vi "populateArrays_sub.vi"(11 "Instance":i32) -> (0 "ENC_VEL_Array":u16[](array[numeric]), 1 "ENC_POS_Array":i32[](array[numeric]), 2 "ADC_Array":dbl[](array[numeric]), 3 "Instance out":i32, 4 "DIN":u16, 6 "Message Count":u32)   [LabVIEW 2022 SP3]
uses:
  LVLib/SADI_FW3.lvlib
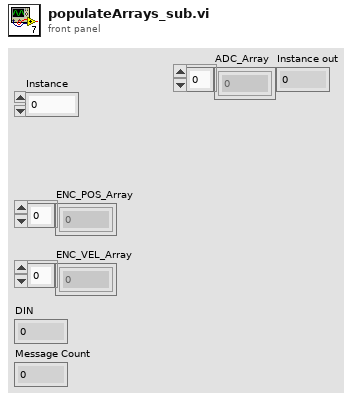
[diagram p1: front panel]
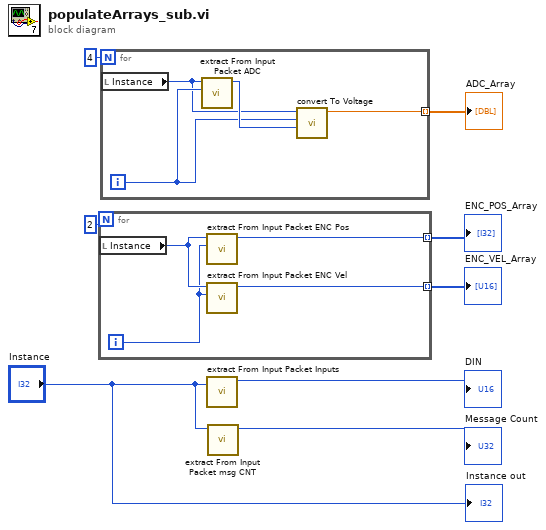
[diagram p0: block diagram]
diagram:
  n1 = for {
    N: 2 -> [_]
    tunnel: [w12] -> w3 mode=indexing
    tunnel: [w11] -> w4 mode=indexing
    i -> [w9]
    n2 = local read "Instance"() -> (w10:i32)
    n3 = call "extract From Input Packet ENC Pos.vi"("channel"=w9, "instance"=w10) -> ("function return"=w12:i32)  [unwired: 9 in]
    n4 = call "extract From Input Packet ENC Vel.vi"("channel"=w9, "instance"=w10) -> ("function return"=w11:i16)  [unwired: 9 in]
  }
  "ENC_VEL_Array" <- w4
  "ENC_POS_Array" <- w3
  n5 = for {
    N: 4 -> [_]
    tunnel: [w13] -> w1 mode=indexing
    i -> [w15]
    n6 = local read "Instance"() -> (w14:i32)
    n7 = call "extract From Input Packet ADC.vi"("channel"=w15, "instance"=w14) -> ("function return"=w16:i16)  [unwired: 9 in]
    n8 = call "convert To Voltage.vi"("value"=w16, "adcCh"=w15, "instance"=w14) -> ("function return"=w13:dbl)  [unwired: 8 in]
  }
  "ADC_Array" <- w1
  n9 = call "extract From Input Packet Inputs.vi"("instance"="Instance") -> ("function return"=→"DIN":u16)  [unwired: 10 in]
  n10 = call "extract From Input Packet msg CNT.vi"("instance"="Instance") -> ("function return"=→"Message Count":u32)  [unwired: 10 in]
  "Instance out" <- "Instance"
